vi "init.vi"(11 "Device Reference in":T2 format="%.0x") -> (0 "error code":i32, 1 "outputs":T1[](array[typedef]) format="%.0x", 2 "inputs":T1[](array[typedef]) format="%.0x", 3 "state":T3)   [LabVIEW 2015, in "Scriptable Model Interface Engine.lvlib"]
uses:
  Scriptable Model Interface Engine.lvlib
  runtime state.ctl
  Shared/model parameters.ctl
  <vilib>/NI Veristand/Custom Device API/Custom Device Item Ref.ctl
  <vilib>/NI Veristand/Custom Device API/Data Reference.ctl
  Shared/model inputs.ctl
  <vilib>/NI Veristand/Custom Device API/Custom Device Channel Type.ctl
  Shared/model outputs.ctl
  <vilib>/NI Veristand/Custom Device API/Data Access Type.ctl
  Shared/Constants.vi
  <vilib>/NI Veristand/Custom Device API/Get Item Property (String).vi
  <vilib>/NI Veristand/Custom Device API/Custom Device API.lvlib
  Shared/Scriptable Model Interface Shared.lvlib
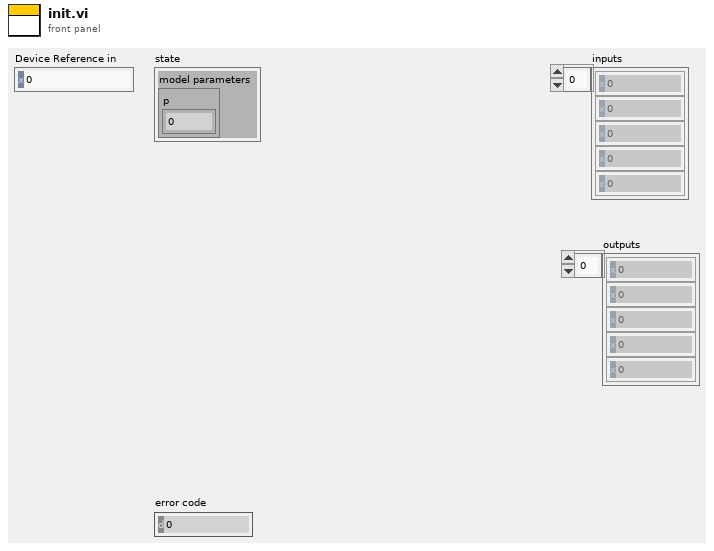
[diagram p1: front panel]
types:
  T1 = typedef "Custom Device API.lvlib/Data Reference.ctl" = i32
  T2 = typedef "Custom Device API.lvlib/Custom Device Item Ref.ctl" = u64
  T3 = typedef "Scriptable Model Interface Engine.lvlib/runtime state.ctl" = cluster{"model parameters":T4}
  T4 = typedef "Scriptable Model Interface Shared.lvlib/model parameters.ctl" = cluster{"p":dbl}
  T5 = typedef "Custom Device API.lvlib/Data Access Type.ctl" = enum16{"Read", "Write"}
  T6 = typedef "Scriptable Model Interface Shared.lvlib/model outputs.ctl" = cluster{"o":dbl}
  T7 = typedef "Custom Device API.lvlib/Custom Device Channel Type.ctl" = enum16{"Input", "Output"}
  T8 = typedef "Scriptable Model Interface Shared.lvlib/model inputs.ctl" = cluster{"i":dbl}
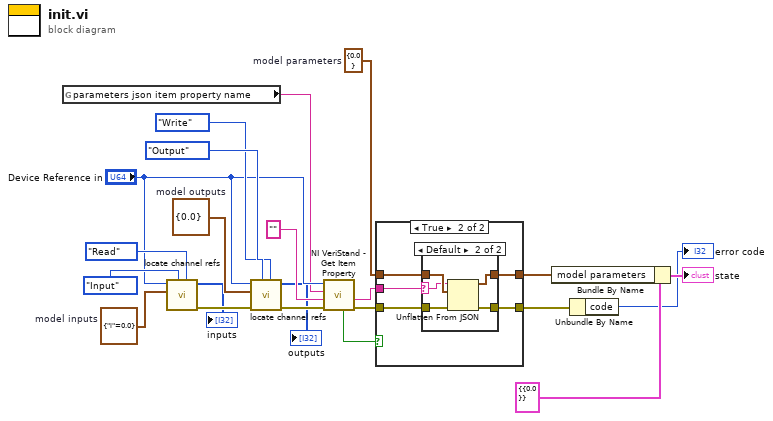
[diagram p0: block diagram]
diagram:
  w21 = T6 {"o"=0.0}  # model outputs
  w8 = T4 {"p"=0.0}  # model parameters
  w20 = T8 {"i"=0.0}  # model inputs
  n1 = global read "Constants.vi" "parameters json item property name"() -> (w7:string)
  n2 = call "locate channel refs.vi"("Access"=Data_Access_Type."Read", "Channel Type"=Custom_Device_Channel_Type."Input", "Variant"=w20, "Device Reference in"="Device Reference in") -> ("error out"=w22:errorcluster, "refs"=→"inputs":T1[])  [unwired: 6 in]
  n3 = call "locate channel refs.vi"("Access"=Data_Access_Type."Write", "Channel Type"=Custom_Device_Channel_Type."Output", "error in"=w22, "Variant"=w21, "Device Reference in"="Device Reference in") -> ("error out"=w11:errorcluster, "refs"=→"outputs":T1[])  [unwired: 5 in]
  n4 = call-poly <vilib>:"NI VeriStand - Get Item Property.vi"("error in (no error)"=w11, "Default Value"="", "Property Name"=w7, "Item Ref in"="Device Reference in") -> ("error out"=w10:errorcluster, "Value"=w4:string, "Found?"=w3:bool)  [unwired: 4 in, 1 out]
  n5 = case shown="True" w3 {
    tunnel: w10 -> [w23 w29]
    tunnel: [w23 w28] -> w9
    tunnel: w8 -> [w24 w27]
    tunnel: [w24 w26] -> w5
    tunnel: w4 -> [_ w25]
    frame False {
    }
    frame True {
      n6 = case shown="Default" w25 {
        selector: w25 -> [_ w32]
        tunnel: w29 -> [w30 w36]
        tunnel: [w30 w35] -> w28
        tunnel: w27 -> [w31 w34]
        tunnel: [w31 w33] -> w26
        frame "" {
        }
        frame Default {
          n7 = Unflatten From JSON(JSON string=w32, type and defaults=w34, error in (no error)=w36) -> (value=w33:T4, error out=w35:errorcluster)  [unwired: 4 in]
        }
      }
    }
  }
  n8 = Bundle By Name(cluster=T3 {"model parameters"={"p"=0.0}} ("state"), "model parameters"=w5) -> (→"state":T3)
  n9 = Unbundle By Name(w9) -> ("code"=→"error code":i32)
